vi "Dialog - Configure Threading.vi"(6 "rxPacket?":bool, 7 "error in (no error)":errorcluster, 9 "threadOptions in":T3 {"pclDecimation" max=16 step=1; "loopPeriod" max=16 step=1; "targetPriority" min=-2 max=16 step=1; "targetProcessor" min=-2 max=16 step=1}, 10 "Packet Ref in":T2 format="%.0x") -> (0 "error out":errorcluster, 2 "threadOptions out":T3 {"pclDecimation" max=16 step=1; "loopPeriod" max=16 step=1; "targetPriority" min=-2 max=16 step=1; "targetProcessor" min=-2 max=16 step=1}, 3 "Packet Ref out":T2 format="%.0x")   [LabVIEW 2023, in "UDP-Custom-Device System Explorer.lvlib"]
uses:
  UDP-Custom-Device System Explorer.lvlib
  Types/Threading/Thread Sync Reference.ctl
  Types/Threading/Thread Configuration.ctl
  Shared/Types/Shared - Thread Management.ctl
  <vilib>/NI VeriStand/Custom Device API/Custom Device Item Ref.ctl
  <vilib>/Utility/miscctls.llb/LVMinMaxIncTypeDef.ctl
  <vilib>/NI VeriStand/Custom Device API/Custom Device Target Type.ctl
  <vilib>/NI VeriStand/Custom Device API/Custom Device API.lvlib
  Shared/UDP-Custom-Device Shared.lvlib
panel:
  in  "Thread Management":T1
  in  "threadSync":T4 caption="Synchronization"
  in  "pclDecimation":u16=1 caption="PCL Decimation" min=1 step=1
  in  "loopPeriod":u32=1 caption="Loop Period (us)" min=1 step=1
  in  "defaultPriority":bool
  in  "targetPriority":i16=1 caption="Priority" min=1 step=1
  in  "defaultProcessor":bool
  in  "targetProcessor":i8 caption="Target Processor" min=-2 max=31 step=1
  in  "Cancel":bool
  in  "OK":bool
  # "Select Packet Threading Options"
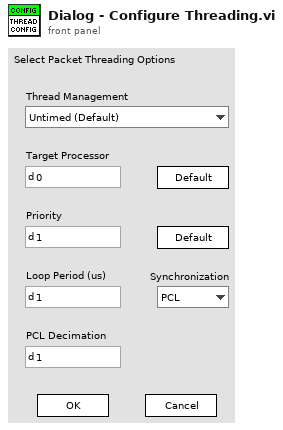
[diagram p1: front panel]
types:
  T1 = typedef "UDP-Custom-Device Shared.lvlib/Shared - Thread Management.ctl" = enum16{"Untimed (Default)", "Timed (High Priority)"}
  T2 = typedef "Custom Device API.lvlib/Custom Device Item Ref.ctl" = u64
  T3 = typedef "UDP-Custom-Device System Explorer.lvlib/Thread Configuration.ctl" = cluster{"targetProcessor":i8, "targetPriority":i16, "Synchronization":T4, "loopPeriod":u32, "pclDecimation":u16, "threadManagement":T1}
  T4 = typedef "UDP-Custom-Device System Explorer.lvlib/Thread Sync Reference.ctl" = enum16{"PCL", "Async"}
  T5 = typedef "Custom Device API.lvlib/Custom Device Target Type.ctl" = enum16{"PharLap", "VxWorks", "Windows", "Linux_32_ARM", "Linux_x64"}
  T6 = typedef "LVMinMaxIncTypeDef.ctl" = cluster{"Minimum":dbl, "Maximum":dbl, "Increment":dbl}
  T7 = enum8{"Enabled", "Disabled", "Disabled and Grayed Out"}
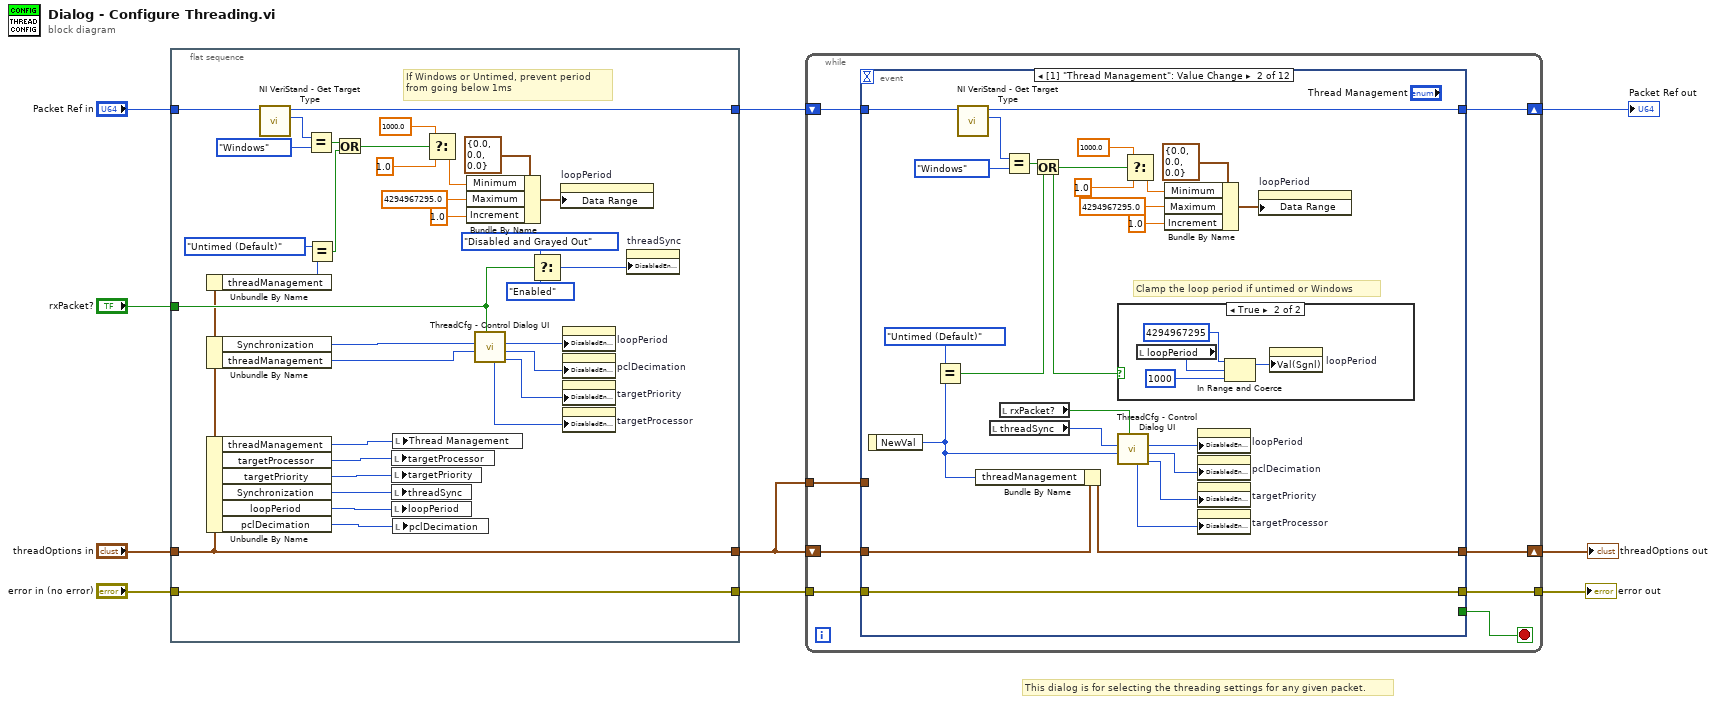
[diagram p0: block diagram]
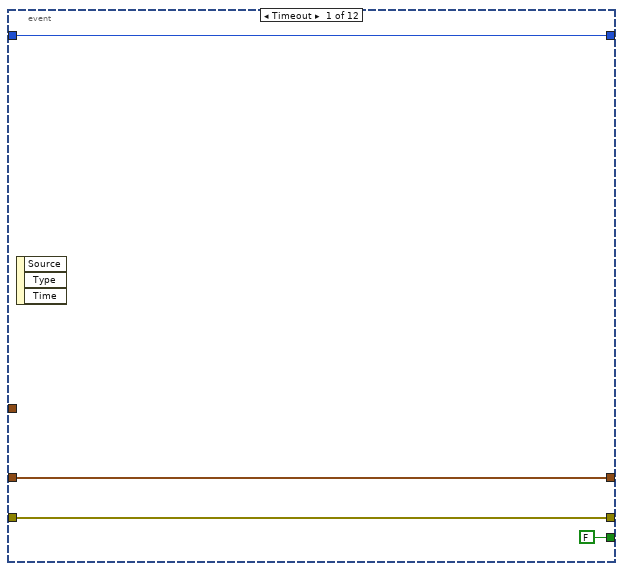
[diagram p2: hidden frame]
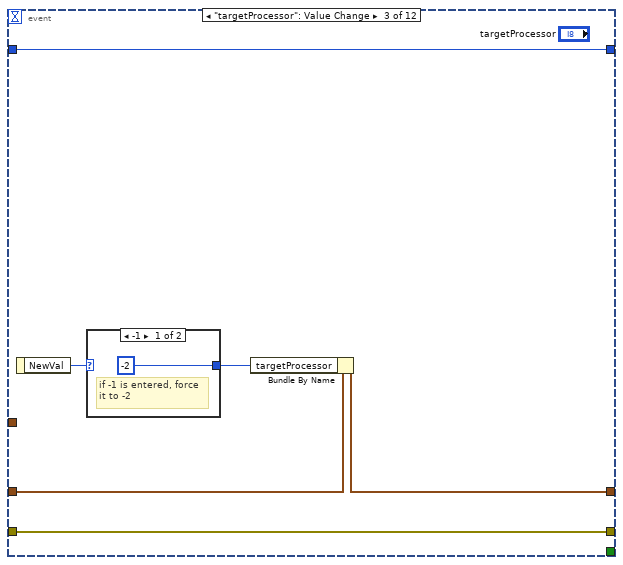
[diagram p4: hidden frame]
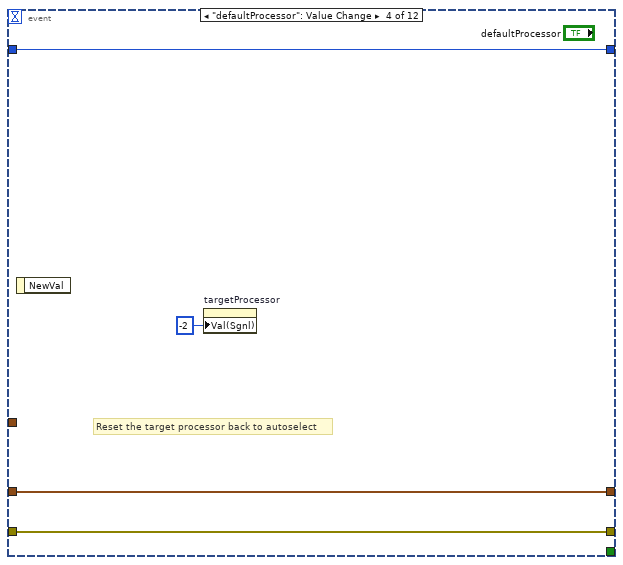
[diagram p6: hidden frame]
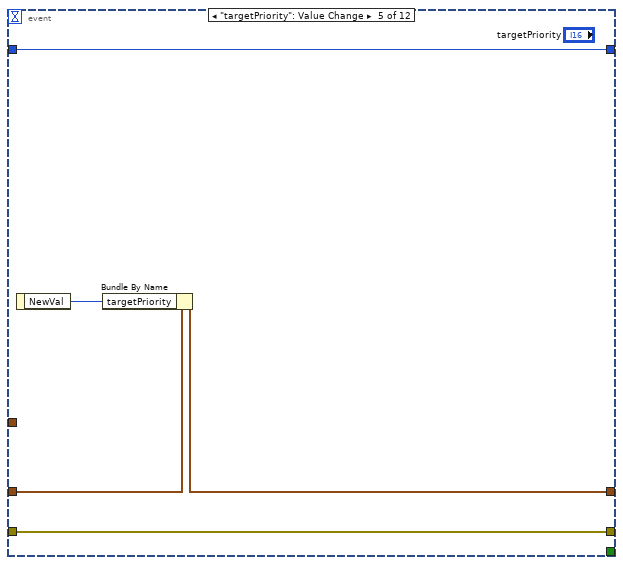
[diagram p7: hidden frame]
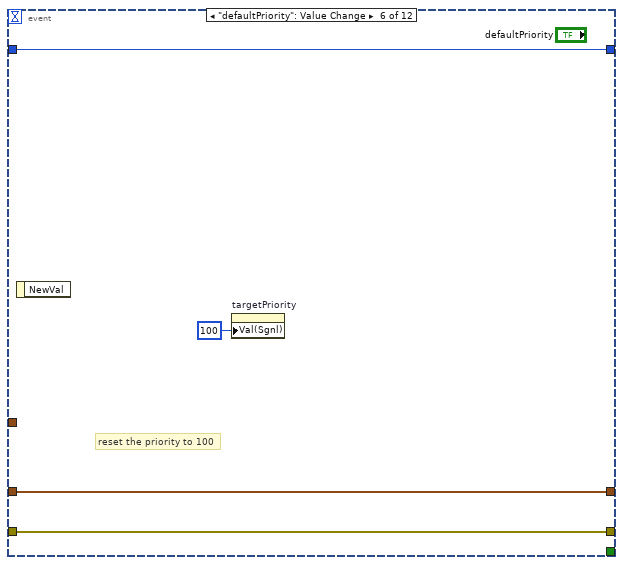
[diagram p8: hidden frame]
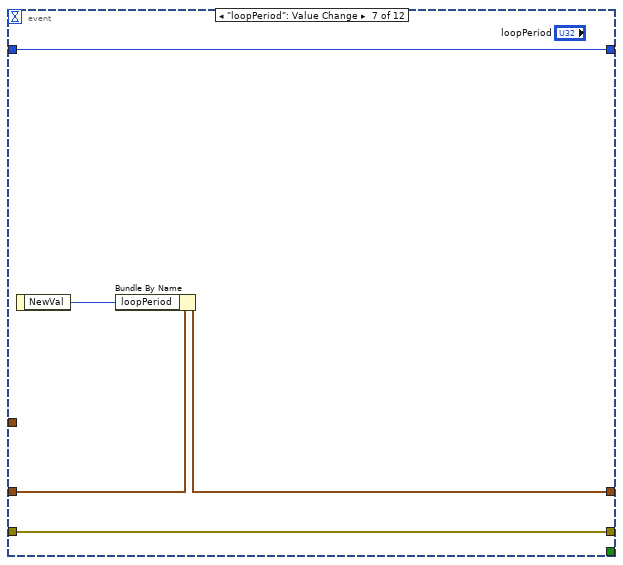
[diagram p9: hidden frame]
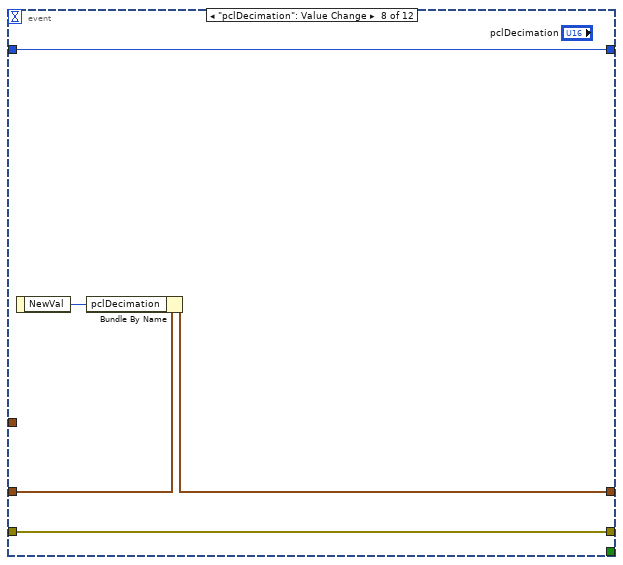
[diagram p10: hidden frame]
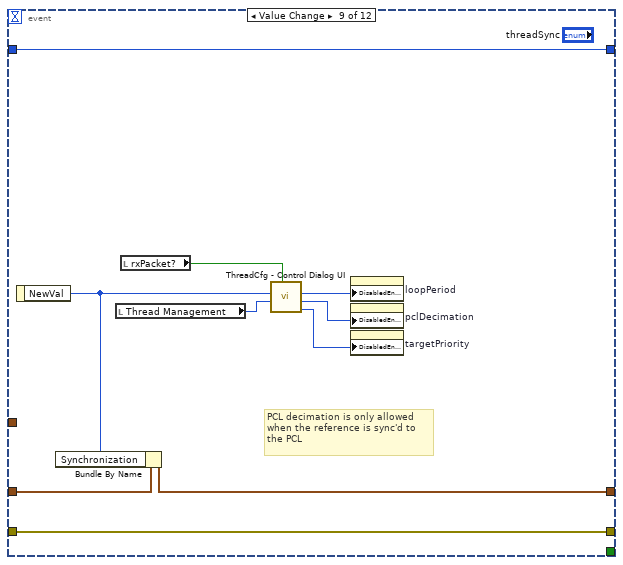
[diagram p11: hidden frame]
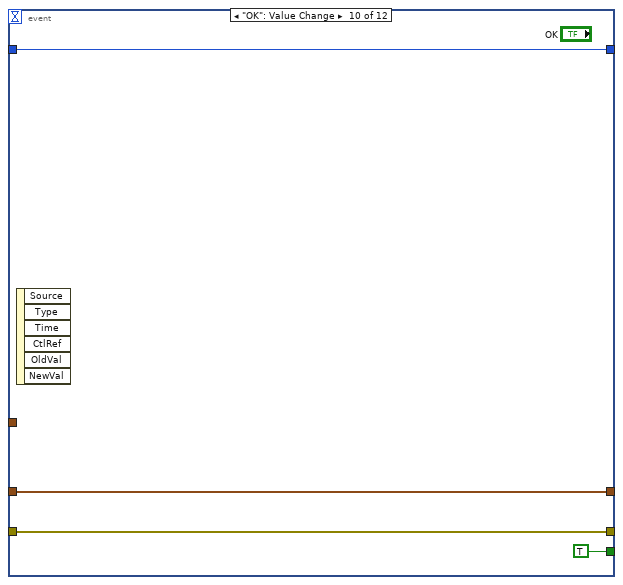
[diagram p12: hidden frame]
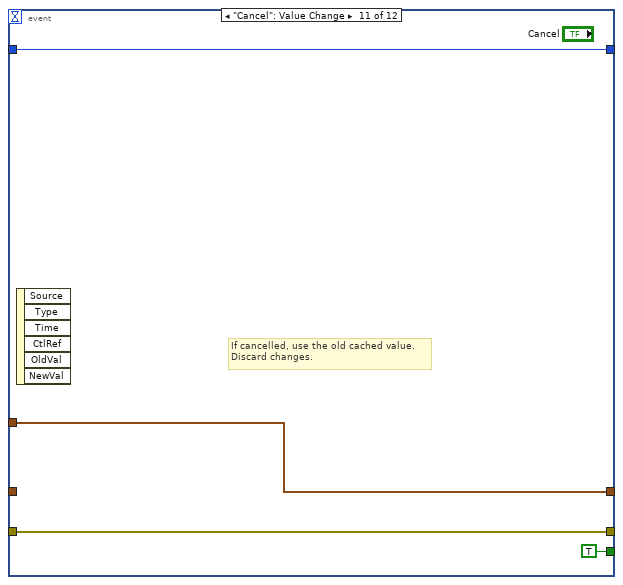
[diagram p13: hidden frame]
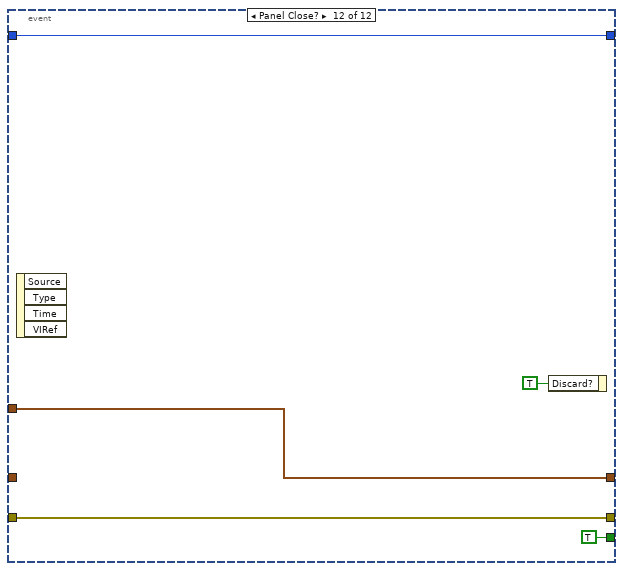
[diagram p14: hidden frame]
diagram:
  # "This dialog is for selecting the threading settings for any given packet."
  n1 = flat-sequence {
    tunnel: "error in (no error)" -> [w44]
    tunnel: [w44] -> w8
    tunnel: "threadOptions in" -> [w19]
    tunnel: [w19] -> w7
    tunnel: "rxPacket?" -> [w32]
    tunnel: [w30] -> w1
    tunnel: "Packet Ref in" -> [w31]
    frame #0 {
      # "If Windows or Untimed, prevent period\nfrom going below 1ms"
      n2 = Unbundle By Name(w19) -> ("threadManagement"=w18:T1)
      n3 = Unbundle By Name(w19) -> ("Synchronization"=w38:T4, "threadManagement"=w20:T1)
      n4 = Unbundle By Name(w19) -> ("threadManagement"=w11:T1, "targetProcessor"=w39:i8, "targetPriority"=w40:i16, "Synchronization"=w41:T4, "loopPeriod"=w42:u32, "pclDecimation"=w43:u16)
      n5 = call <vilib>:"NI VeriStand - Get Target Type.vi"("Item Ref in"=w31) -> ("Target Type"=w29:T5, "Item Ref out"=w30:T2)  [unwired: 8 in, 1 out]
      n6 = Equal?(x=w29, y=Custom_Device_Target_Type."Windows") -> (x = y?=w15:bool)
      n7 = Equal?(x=Shared_-_Thread_Management."Untimed (Default)", y=w18) -> (x = y?=w16:bool)
      n8 = Or(x=w15, y=w16) -> (x .or. y?=w14:bool)
      n9 = local write "targetProcessor"(w39) -> ()
      n10 = local write "targetPriority"(w40) -> ()
      n11 = local write "threadSync"(w41) -> ()
      n12 = local write "loopPeriod"(w42) -> ()
      n13 = local write "Thread Management"(w11) -> ()
      n14 = local write "pclDecimation"(w43) -> ()
      n15 = Select(t=1000.0 ("Minimum"), s=w14, f=1.0 ("Minimum")) -> (s? t:f=w21:dbl)
      n16 = Bundle By Name(cluster=T6 {"Minimum"=0.0, "Maximum"=0.0, "Increment"=0.0} ("Data Entry Limits"), "Minimum"=w21, "Maximum"=4294967295.0, "Increment"=1.0 ("Minimum")) -> (w26:T6)
      n17 = call "ThreadCfg - Control Dialog UI.vi"("rxPacket?"=w32, "threadManagement"=w20, "threadPeriodRef"=w38) -> ("priorityState"=w13:T7, "pclDecimationState"=w36:T7, "loopPeriodState"=w37:T7, "processorState"=w12:T7)  [unwired: 5 in]
      n18 = Select(t=T7."Disabled and Grayed Out" ("Disabled"), s=w32, f=T7."Enabled" ("Disabled")) -> (s? t:f=w33:T7)
      n19 = property on="loopPeriod" class="DigNum (strict)"("Data Range"=w26) -> ()  [unwired: 2 in, 2 out]
      n20 = property on="loopPeriod" class="DigNum (strict)"("DisabledEnum"=w37) -> ()  [unwired: 2 in, 2 out]
      n21 = property on="pclDecimation" class="DigNum (strict)"("DisabledEnum"=w36) -> ()  [unwired: 2 in, 2 out]
      n22 = property on="targetPriority" class="DigNum (strict)"("DisabledEnum"=w13) -> ()  [unwired: 2 in, 2 out]
      n23 = property on="targetProcessor" class="DigNum (strict)"("DisabledEnum"=w12) -> ()  [unwired: 2 in, 2 out]
      n24 = property on="threadSync" class="Enum (strict)"("DisabledEnum"=w33) -> ()  [unwired: 2 in, 2 out]
    }
  }
  n25 = while {
    tunnel: w8 -> [w50]
    shift-right: [w47] -> w5
    shift-left: w7 -> [w51]
    tunnel: w7 -> [w52]
    tunnel: [w48] -> w6
    shift-right: [w46] -> w2
    shift-left: w1 -> [w45]
    stop <- w49 stop-if-true
    n26 = event shown="[1] \"Thread Management\": Value Change" {
      selector: _ -> [_ _ _ _ _ _ _ _ _ _ _ _]
      dyn-events: _ -> [_ _ _ _ _ _ _ _ _ _ _ _]
      timeout: _ -> [_ _ _ _ _ _ _ _ _ _ _ _]
      tunnel: w52 -> [_ _ _ _ _ _ _ _ _ _ w133 w138]
      tunnel: w51 -> [w54 w80 w90 w96 w100 w105 w110 w115 w125 w129 _ _]
      tunnel: w50 -> [w55 w81 w91 w97 w102 w106 w111 w116 w126 w130 w134 w139]
      tunnel: [FALSE _ _ _ _ _ _ _ _ TRUE TRUE TRUE] -> w49
      tunnel: [w55 w81 w91 w97 w102 w106 w111 w116 w126 w130 w134 w139] -> w48
      tunnel: [w54 w79 w89 w96 w99 w105 w109 w114 w124 w129 w133 w138] -> w47
      tunnel: [w53 w61 w86 w94 w98 w103 w107 w112 w117 w127 w131 w135] -> w46
      tunnel: w45 -> [w53 w62 w86 w94 w98 w103 w107 w112 w117 w127 w131 w135]
      event Timeout {
        n27 = event-data() -> ()  [unwired: 1 in, 3 out]
      }
      event Value Change {
        # "Clamp the loop period if untimed or Windows"
        n28 = event-data() -> ("NewVal"=w74:T1)  [unwired: 1 in]
        n29 = Equal?(x=Shared_-_Thread_Management."Untimed (Default)", y=w74) -> (x = y?=w63:bool)
        n30 = call <vilib>:"NI VeriStand - Get Target Type.vi"("Item Ref in"=w62) -> ("Target Type"=w64:T5, "Item Ref out"=w61:T2)  [unwired: 8 in, 1 out]
        n31 = Bundle By Name(cluster=w80, "threadManagement"=w74) -> (w79:T3)
        n32 = local read "threadSync"() -> (w60:T4)
        n33 = local read "rxPacket?"() -> (w77:bool)
        n34 = Equal?(x=w64, y=Custom_Device_Target_Type."Windows") -> (x = y?=w73:bool)
        n35 = Or(x=w73, y=w63) -> (x .or. y?=w57:bool)
        n36 = case shown="True" w57 {
          frame False {
          }
          frame True {
            n37 = local read "loopPeriod"() -> (w84:u32)
            n38 = In Range and Coerce(upper limit=u32 4294967295 ("Maximum"), x=w84, lower limit=u32 1000 ("loopPeriod")) -> (coerced(x)=w83:u32)  [unwired: 1 out]
            n39 = property on="loopPeriod" class="DigNum (strict)"("Val(Sgnl)"=w83) -> ()  [unwired: 2 in, 2 out]
          }
        }
        n40 = call "ThreadCfg - Control Dialog UI.vi"("rxPacket?"=w77, "threadManagement"=w74, "threadPeriodRef"=w60) -> ("priorityState"=w59:T7, "pclDecimationState"=w75:T7, "loopPeriodState"=w76:T7, "processorState"=w58:T7)  [unwired: 5 in]
        n41 = Select(t=1000.0 ("Minimum"), s=w57, f=1.0 ("Minimum")) -> (s? t:f=w72:dbl)
        n42 = Bundle By Name(cluster=T6 {"Minimum"=0.0, "Maximum"=0.0, "Increment"=0.0} ("Data Entry Limits"), "Minimum"=w72, "Maximum"=4294967295.0, "Increment"=1.0 ("Minimum")) -> (w67:T6)
        n43 = property on="loopPeriod" class="DigNum (strict)"("DisabledEnum"=w76) -> ()  [unwired: 2 in, 2 out]
        n44 = property on="pclDecimation" class="DigNum (strict)"("DisabledEnum"=w75) -> ()  [unwired: 2 in, 2 out]
        n45 = property on="targetPriority" class="DigNum (strict)"("DisabledEnum"=w59) -> ()  [unwired: 2 in, 2 out]
        n46 = property on="targetProcessor" class="DigNum (strict)"("DisabledEnum"=w58) -> ()  [unwired: 2 in, 2 out]
        n47 = property on="loopPeriod" class="DigNum (strict)"("Data Range"=w67) -> ()  [unwired: 2 in, 2 out]
      }
      event "targetProcessor": Value Change {
        n48 = event-data() -> ("NewVal"=w88:i8)  [unwired: 1 in]
        n49 = case shown="-1" w88 {
          selector: w88 -> [_ w93]
          tunnel: [i8 -2 w93] -> w87
          frame -1 {
            # "if -1 is entered, force\nit to -2"
          }
          frame Default {
          }
        }
        n50 = Bundle By Name(cluster=w90, "targetProcessor"=w87) -> (w89:T3)
      }
      event "defaultProcessor": Value Change {
        # "Reset the target processor back to autoselect"
        n51 = event-data() -> ()  [unwired: 1 in, 1 out]
        n52 = property on="targetProcessor" class="DigNum (strict)"("Val(Sgnl)"=i8 -2 ("Value (Signaling)")) -> ()  [unwired: 2 in, 2 out]
      }
      event "targetPriority": Value Change {
        n53 = event-data() -> ("NewVal"=w101:i16)  [unwired: 1 in]
        n54 = Bundle By Name(cluster=w100, "targetPriority"=w101) -> (w99:T3)
      }
      event "defaultPriority": Value Change {
        # "reset the priority to 100"
        n55 = event-data() -> ()  [unwired: 1 in, 1 out]
        n56 = property on="targetPriority" class="DigNum (strict)"("Val(Sgnl)"=i16 100 ("Value (Signaling)")) -> ()  [unwired: 2 in, 2 out]
      }
      event "loopPeriod": Value Change {
        n57 = event-data() -> ("NewVal"=w108:u32)  [unwired: 1 in]
        n58 = Bundle By Name(cluster=w110, "loopPeriod"=w108) -> (w109:T3)
      }
      event "pclDecimation": Value Change {
        n59 = event-data() -> ("NewVal"=w113:u16)  [unwired: 1 in]
        n60 = Bundle By Name(cluster=w115, "pclDecimation"=w113) -> (w114:T3)
      }
      event Value Change {
        # "PCL decimation is only allowed\nwhen the reference is sync'd to\nthe PCL"
        n61 = event-data() -> ("NewVal"=w122:T4)  [unwired: 1 in]
        n62 = Bundle By Name(cluster=w125, "Synchronization"=w122) -> (w124:T3)
        n63 = local read "Thread Management"() -> (w119:T1)
        n64 = local read "rxPacket?"() -> (w123:bool)
        n65 = call "ThreadCfg - Control Dialog UI.vi"("rxPacket?"=w123, "threadManagement"=w119, "threadPeriodRef"=w122) -> ("priorityState"=w118:T7, "pclDecimationState"=w120:T7, "loopPeriodState"=w121:T7)  [unwired: 5 in, 1 out]
        n66 = property on="loopPeriod" class="DigNum (strict)"("DisabledEnum"=w121) -> ()  [unwired: 2 in, 2 out]
        n67 = property on="pclDecimation" class="DigNum (strict)"("DisabledEnum"=w120) -> ()  [unwired: 2 in, 2 out]
        n68 = property on="targetPriority" class="DigNum (strict)"("DisabledEnum"=w118) -> ()  [unwired: 2 in, 2 out]
      }
      event "OK": Value Change {
        n69 = event-data() -> ()  [unwired: 1 in, 6 out]
      }
      event "Cancel": Value Change {
        # "If cancelled, use the old cached value.\nDiscard changes."
        n70 = event-data() -> ()  [unwired: 1 in, 6 out]
      }
      event Panel Close? {
        n71 = event-data() -> ()  [unwired: 1 in, 4 out]
        n72 = event-data("Discard?"=TRUE) -> ()  [unwired: 1 in, 1 out]
      }
    }
  }
  "error out" <- w6
  "threadOptions out" <- w5
  "Packet Ref out" <- w2
